vi "Update Data.vi"(8 "error in":errorcluster, 10 "Data":cluster{"Numeric":i32}, 11 "CutomOOB_Tx in":refnum<class "CIFCustomOOB_Tx.lvclass">) -> (0 "error out":errorcluster, 3 "CutomOOB_Tx out":refnum<class "CIFCustomOOB_Tx.lvclass">)   [LabVIEW 2021, in "CIFCustomOOB_Tx.lvclass"]
uses:
  CIFCustomOOB_Tx.lvclass
  CIFCustomOOB_Tx.lvclass/CIFCustomOOB_Tx.ctl
  CIFUtilities/CIFOutOfBand/CIFOutOfBand.lvclass
  Typedef/OOB Commands.ctl
  Typedef/Payload.ctl
  D:/dev/CIF-LVCore/src/CIFUtilities/CIFOutOfBand/CIFOutOfBand.lvclass
  D:/dev/CIF-LVCore/src/CIFTemplatePlugin/OOB/OOB_Tx/CIFCustomOOB_Tx.lvclass
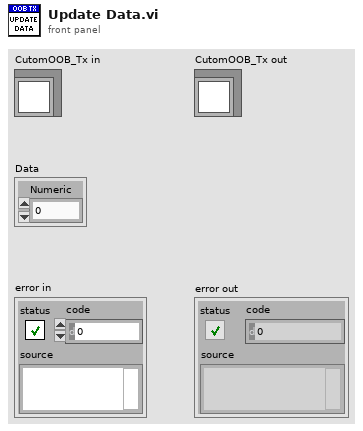
[diagram p1: front panel]
types:
  T1 = typedef "CIFCustomOOB_Tx.lvclass/Payload.ctl" = cluster{"Data":cluster{"Numeric":i32}}
  T2 = typedef "CIFCustomOOB_Tx.lvclass/OOB Commands.ctl" = enum8{"Update Data"}
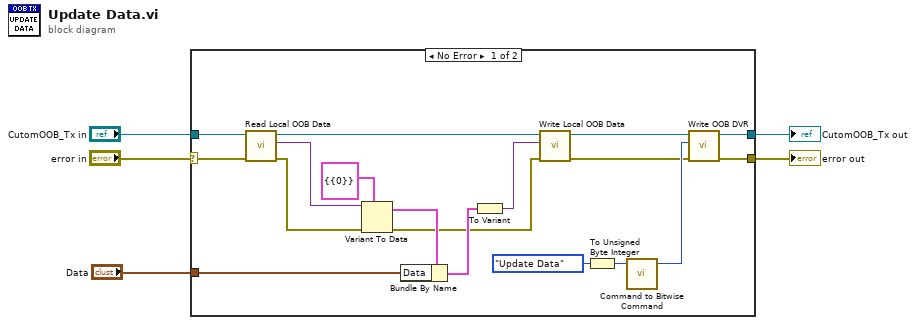
[diagram p0: block diagram]
diagram:
  n1 = case shown="No Error" "error in" {
    selector: "error in" -> [w7 w25]
    tunnel: [w22 w25] -> w4
    tunnel: "CutomOOB_Tx in" -> [w8 w24]
    tunnel: [w23 w24] -> w2
    tunnel: "Data" -> [w6 _]
    frame No Error {
      n2 = call "Read Local OOB Data.vi"("error in"=w7, "OOB in"=w8) -> ("error out"=w14:errorcluster, "Local OOB Data"=w17:variant, "OOB out"=w18:refnum<class "CIFCustomOOB_Tx.lvclass">)  [unwired: 7 in]
      n3 = Variant To Data(error in=w14, type=T1 {"Data"={"Numeric"=0}} ("Template Payload"), Variant=w17) -> (data=w15:T1, error out=w11:errorcluster)
      n4 = Bundle By Name(cluster=w15, "Data"=w6) -> (w13:T1)
      n5 = To Variant(anything=w13) -> (Variant=w12:variant)
      n6 = call "Write Local OOB Data.vi"("error in"=w11, "Local OOB Data"=w12, "OOB in"=w18) -> ("error out"=w9:errorcluster, "OOB out"=w10:refnum<class "CIFCustomOOB_Tx.lvclass">)  [unwired: 7 in]
      n7 = To Unsigned Byte Integer(number=OOB_Commands."Update Data" ("OOB Main Commands")) -> (unsigned 8bit integer=w21:u8)
      n8 = call "Command to Bitwise Command.vi"("OOB Command"=w21) -> ("bit command"=w20:u64)  [unwired: 3 in]
      n9 = call "Write OOB DVR.vi"("error in"=w9, "Commands (bitwise)"=w20, "OOB in"=w10) -> ("error out"=w22:errorcluster, "OOB out"=w23:refnum<class "CIFCustomOOB_Tx.lvclass">)  [unwired: 7 in]
    }
    frame Error {
    }
  }
  "error out" <- w4
  "CutomOOB_Tx out" <- w2
